vi "fc_test.vi"() -> ()   [LabVIEW 2011]
panel:
  out "Limit fail":bool
  out "Fit characteristics":string[][](table)
  in  "Poly coeffs":string[][](table)
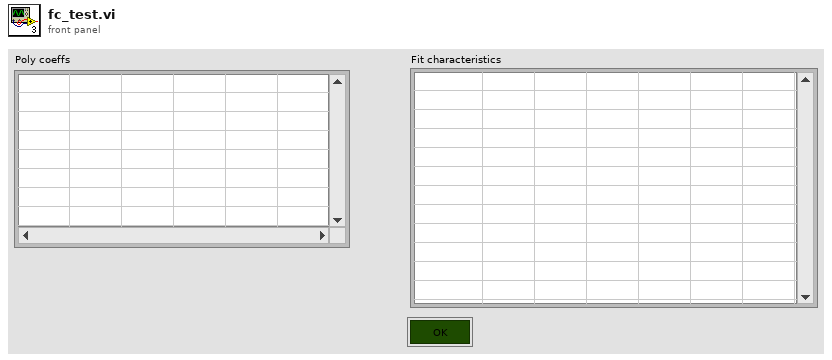
[diagram p1: front panel]
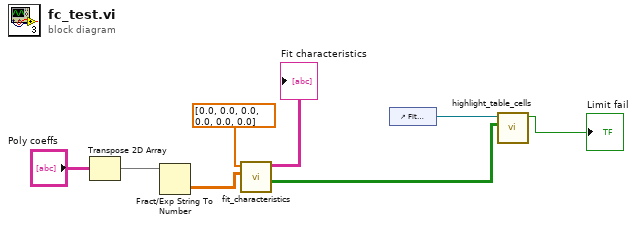
[diagram p0: block diagram]
diagram:
  n1 = Transpose 2D Array(2D array="Poly coeffs") -> (transposed array=w6:string[][])
  n2 = Fract/Exp String To Number(string=w6) -> (number=w5:dbl[][])  [unwired: 3 in, 1 out]
  n3 = call "fit_characteristics.vi"("Polynomial Coefficients"=w5, "Residue"=dbl[] [0.0, 0.0, 0.0, 0.0, 0.0, 0.0]) -> ("Limit fail"=w8:bool[][], "Fit characteristics"=→"Fit characteristics":string[][])  [unwired: 8 in]
  n4 = control-ref of="Fit characteristics"() -> (w2:refnum<vi>)
  n5 = call "highlight_table_cells.vi"("Limit fail"=w8, "Table in"=w2) -> ("Some limit fail"=→"Limit fail":bool)  [unwired: 9 in]
